vi "CTL_SpecCheck.vi"(8 "Level in":dbl=3.635000000000013 format="%#_13g", 11 "Spec Range In":T1={"Specs"=[3.735, 3.635, 4.085, 1011.0, 989.0, 910.0, 890.0], "LUT Status"={"ChA/!ChB"=FALSE, "Drain/!Fill"=FALSE, "In Range?"=TRUE, "Switch Range?"=FALSE, "Measure R?"=FALSE, "Vaild R?"=TRUE, "Index(n)"=10, "Index(n-1)"=9, "Index Max"=13}}) -> (3 "Spec Range Out":T1={"Specs"=[3.735, 3.635, 4.085, 1011.0, 989.0, 910.0, 890.0], "LUT Status"={"ChA/!ChB"=FALSE, "Drain/!Fill"=FALSE, "In Range?"=TRUE, "Switch Range?"=TRUE, "Measure R?"=FALSE, "Vaild R?"=FALSE, "Index(n)"=10, "Index(n-1)"=9, "Index Max"=13}})   [LabVIEW 2024]
uses:
  Control Definitions/Def Spec RNG.ctl
  Control Definitions/Ded LUT_Status.ctl
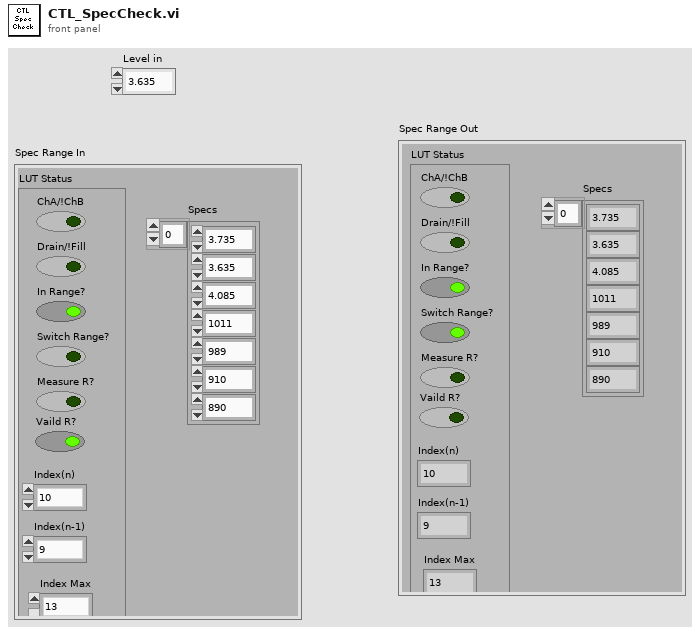
[diagram p1: front panel]
types:
  T1 = typedef "Def Spec RNG.ctl" = cluster{"Specs":dbl[], "LUT Status":T2}
  T2 = typedef "Ded LUT_Status.ctl" = cluster{"ChA/!ChB":bool, "Drain/!Fill":bool, "In Range?":bool, "Switch Range?":bool, "Measure R?":bool, "Vaild R?":bool, "Index(n)":i32, "Index(n-1)":i32, "Index Max":i32}
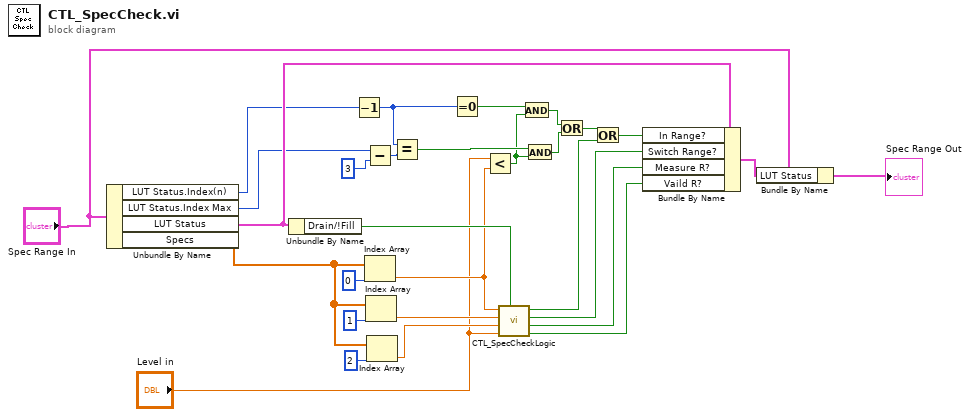
[diagram p0: block diagram]
diagram:
  n1 = Unbundle By Name("Spec Range In") -> ("LUT Status.Index(n)"=w9:i32, "LUT Status.Index Max"=w10:i32, "LUT Status"=w13:T2, "Specs"=w29:dbl[])
  n2 = Unbundle By Name(w13) -> ("Drain/!Fill"=w7:bool)
  n3 = Decrement(x=w9) -> (x-1=w27:i32)
  n4 = Subtract(x=w10, y=3) -> (x-y=w22:i32)
  n5 = Index Array(array=w29, index=0) -> (element=w6:dbl)
  n6 = Index Array(array=w29, index=1) -> (element=w5:dbl)
  n7 = Index Array(array=w29, index=2) -> (element=w4:dbl)
  n8 = Equal?(x=w27, y=w22) -> (x = y?=w17:bool)
  n9 = Equal To 0?(x=w27) -> (x = 0?=w18:bool)
  n10 = Less?(x="Level in", y=w6) -> (x < y?=w3:bool)
  n11 = call "CTL_SpecCheckLogic.vi"("Drain!Fill In"=w7, "Level in"="Level in", "Spec Hi(n+1)"=w4, "Spec Lo (n)"=w5, "Spec Hi (n)"=w6) -> ("Vaild R?"=w8:bool, "Measure R?"=w1:bool, "Switch Range?"=w26:bool, "In Range?"=w24:bool)  [unwired: 2 in, 1 out]
  n12 = And(x=w18, y=w3) -> (x .and. y?=w20:bool)
  n13 = And(x=w17, y=w3) -> (x .and. y?=w19:bool)
  n14 = Or(x=w20, y=w19) -> (x .or. y?=w23:bool)
  n15 = Or(x=w23, y=w24) -> (x .or. y?=w25:bool)
  n16 = Bundle By Name(cluster=w13, "In Range?"=w25, "Switch Range?"=w26, "Measure R?"=w1, "Vaild R?"=w8) -> (w28:T2)
  n17 = Bundle By Name(cluster="Spec Range In", "LUT Status"=w28) -> (→"Spec Range Out":T1)
